vi "_Close Communications_libESP301.vi"(0 "Instrument Channel":string="GPIB/0:4,0", 11 "error in (no error)":errorcluster) -> (15 "error out":errorcluster)   [LabVIEW 2019, in "Newport ESP301.lvlib"]
doc: "This VI closes the I/O interface with the instrument."
uses:
  Newport ESP301.lvlib
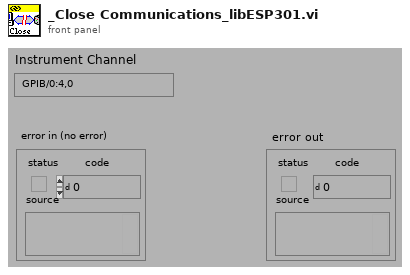
[diagram p1: front panel]
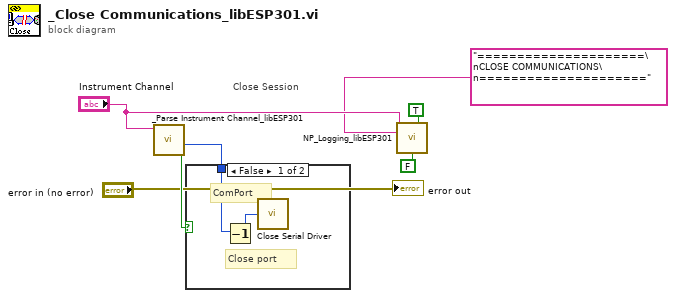
[diagram p0: block diagram]
diagram:
  # "Close Session"
  n1 = call "_Parse Instrument Channel_libESP301.vi"("Instrument Channel"="Instrument Channel") -> ("T - GPIB, F - RS232"=w6:bool, "Hardware Address"=w7:i32)  [unwired: 6 in, 3 out]
  n2 = case shown="False" w6 {
    tunnel: w7 -> [w8 _]
    frame False {
      # "ComPort"
      # "Close port"
      n3 = Decrement(x=w8) -> (x-1=w9:i32)
      n4 = call <vilib>:"Close Serial Driver.vi"("port number"=w9) -> ()  [unwired: 1 out]
    }
    frame True {
    }
  }
  n5 = call "NP_Logging_libESP301.vi"("Instrument Channel"="Instrument Channel", "Generic Strings"=TRUE, "String 1 {Write} (in)"="=====================\nCLOSE COMMUNICATIONS\n=====================", "String 2 Enable (T)"=FALSE) -> ()  [unwired: 8 in, 4 out]
  "error out" <- "error in (no error)"
